vi "Save User Apps.vi"(8 "error in (no error)":errorcluster, 11 "picoG in":refnum<class "picoG.lvclass">) -> (0 "error out":errorcluster, 3 "picoG out":refnum<class "picoG.lvclass">)   [LabVIEW 2020, in "PicoG-App.lvlib" / "picoG.lvclass"]
uses:
  picoG.lvclass
  picoG.lvclass/picoG.ctl
  <vilib>/Utility/config.llb/Write Key (I32).vi
  <vilib>/Utility/config.llb/Write Key (Path).vi
  AppListPanel/AppListPanel.lvclass
  PicoG-App.lvlib
  <vilib>/Utility/config.llb/NI_LVConfig.lvlib
  ViaApp/ViaApp.lvclass
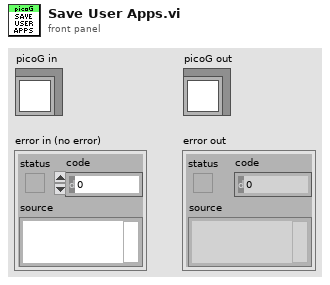
[diagram p1: front panel]
types:
  T1 = typedef "PicoG-App.lvlib/Paths.ctl" = cluster{"User picoG":path, "System picoG":path, "User Config":path, "System Config":path}
  T2 = typedef "NI_LVConfig.lvlib/Config Data RefNum.ctl" = refnum<k1>
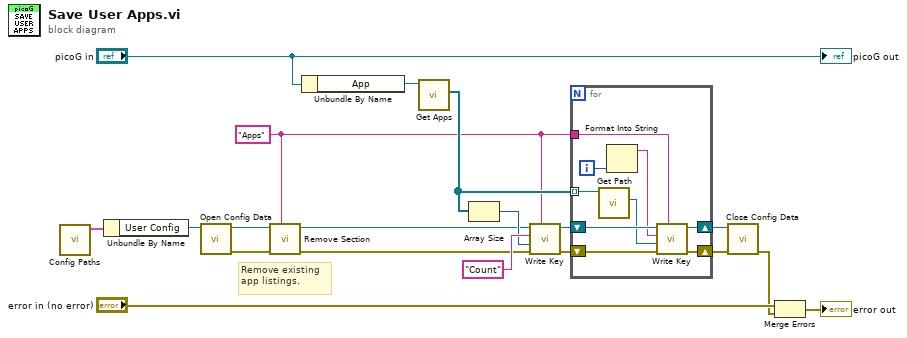
[diagram p0: block diagram]
diagram:
  w5 = "Apps" ("section")
  # "Remove existing app listings."
  n1 = call "Config Paths.vi"() -> ("Paths"=w16:T1)  [unwired: 8 in, 3 out]
  n2 = Unbundle By Name(w16) -> ("User Config"=w15:path)
  n3 = call <vilib>:"Open Config Data.vi"("configuration file path"=w15) -> ("error out"=w8:errorcluster, "refnum"=w9:T2)  [unwired: 8 in, 1 out]
  n4 = call <vilib>:"Remove Section.vi"("section"=w5, "error in (no error)"=w8, "refnum"=w9) -> ("error out"=w6:errorcluster, "refnum out"=w7:T2)  [unwired: 6 in, 1 out]
  n5 = Unbundle By Name("picoG in") -> ("App"=w17:refnum<class "AppListPanel.lvclass">)
  n6 = call "Get Apps.vi"("AppListPanel in"=w17) -> ("Apps"=w14:refnum<class "ViaApp.lvclass">[])  [unwired: 8 in, 2 out]
  n7 = Array Size(array=w14) -> (size(s)=w10:i32)
  n8 = call-poly <vilib>:"Write Key.vi"("section"=w5, "error in (no error)"=w6, "value"=w10, "key"="Count", "refnum"=w7) -> ("error out"=w12:errorcluster, "refnum out"=w13:T2)  [unwired: 4 in, 1 out]
  n9 = for {
    shift-right: [w22] -> w4
    shift-left: w13 -> [w28]
    shift-right: [w21] -> w3
    shift-left: w12 -> [w27]
    tunnel: w14 -> [w24] mode=indexing
    tunnel: w5 -> [w20]
    i -> [w26]
    n10 = call "Get Path.vi"("ViaApp in"=w24) -> ("Path"=w23:path)  [unwired: 8 in, 2 out]
    n11 = Format Into String(w26) -> (resulting string=w25:string)  [unwired: 3 in, 1 out]
    n12 = call-poly <vilib>:"Write Key.vi"("section"=w20, "error in (no error)"=w27, "value"=w23, "key"=w25, "refnum"=w28) -> ("error out"=w21:errorcluster, "refnum out"=w22:T2)  [unwired: 4 in, 1 out]
  }
  n13 = call <vilib>:"Close Config Data.vi"("error in (no error)"=w3, "refnum"=w4) -> ("error out"=w1:errorcluster)  [unwired: 8 in, 1 out]
  n14 = Merge Errors("error in (no error)", w1) -> (→"error out":errorcluster)
  "picoG out" <- "picoG in"
